vi "Read Enable.vi"(8 "error in (no error)":errorcluster, 11 "DAQ HVPS in":refnum<class "DAQ HVPS.lvclass">) -> (0 "error out":errorcluster, 2 "Enable":refnum<k21>, 3 "DAQ HVPS out":refnum<class "DAQ HVPS.lvclass">)   [LabVIEW 2013, in "DAQ HVPS.lvclass"]
uses:
  DAQ HVPS.lvclass
  DAQ HVPS.lvclass/DAQ HVPS.ctl
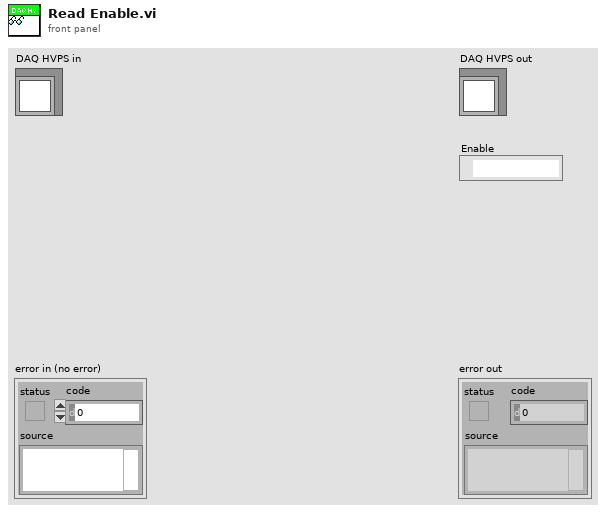
[diagram p1: front panel]
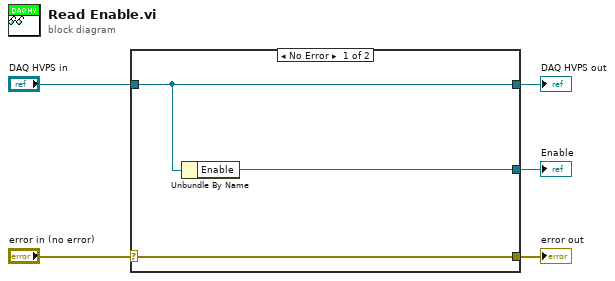
[diagram p0: block diagram]
diagram:
  n1 = case shown="No Error" "error in (no error)" {
    selector: "error in (no error)" -> [w8 w9]
    tunnel: [w8 w9] -> w4
    tunnel: [w7 w10] -> w2
    tunnel: "DAQ HVPS in" -> [w7 w10]
    tunnel: [w6 _] -> w1
    frame No Error {
      n2 = Unbundle By Name(w7) -> ("Enable"=w6:refnum<k21>)
    }
    frame Error {
    }
  }
  "error out" <- w4
  "DAQ HVPS out" <- w2
  "Enable" <- w1
